vi "API Usage Examples.vi"() -> ()   [LabVIEW 2024, in "serenial.io-ase.example.lvlib"]
doc: "<B>A range of API usage examples for different scenarios.</B>"
uses:
  serenial.io-ase.example.lvlib
  serenial.io-ase/ase/ase.lvclass/ase.ctl
  Example Custom Regex/Example Custom Regex.lvclass
  serenial.io-ase/ase/Standard Output.ctl
  serenial.io-ase/ase/Did Exit.ctl
  serenial.io-ase/ase/Event References.ctl
  serenial.io-ase/ase/Standard Error.ctl
  serenial.io-ase/ase/Start Call (Command).vi
  serenial.io-ase/ase/Write Line to Std In .vi
  serenial.io-ase/ase/Start Call (Exe-Args).vi
  serenial.io-ase/ase/Start Call (Internal).vi
  serenial.io-ase/ase/Merge Call Library Errors.vi
  serenial.io-ase/ase/Write Data to Std In.vi
  serenial.io-ase/ase/Error Invalid ASE Handle.vi
  serenial.io-ase/ase/Error Empty Executable Name.vi
  serenial.io-ase/ase/Check Shared Library Version.vi
  serenial.io-ase/ase/Trim Whitespace.vi
  serenial.io-ase/ase/Error Internal Library Implementation Error.vi
  Example Custom ID/Example Custom ID.lvclass
  <vilib>/Utility/error.llb/Error Cluster From Error Code.vi
  serenial.io-ase/configuration/configuration.lvclass
  serenial.io-ase/ase/ase.lvclass
  C:/Users/marc/code/sift-streaming/labview/Sift/Dependencies/asynchronous-system-exec-v2.0.0/serenial.io-ase/configuration/configuration.lvclass
  C:/Users/marc/code/sift-streaming/labview/Sift/Dependencies/asynchronous-system-exec-v2.0.0/serenial.io-ase.example/Example Custom ID/Example Custom ID.lvclass
  C:/Users/marc/code/sift-streaming/labview/Sift/Dependencies/asynchronous-system-exec-v2.0.0/serenial.io-ase.example/Example Custom Regex/Example Custom Regex.lvclass
panel:
  out "Exit Code":i32
  out "error out":errorcluster
  out "Exit Code":i32
  out "error out":errorcluster
  out "Std Out":string caption="Std Out (regex split on numeric)"
  out "Exit Code":i32
  out "error out":errorcluster
  out "Std Out":string
  out "error out":errorcluster
  out "Std Out":string
  out "error out":errorcluster
  out "Std Out":string
  out "Exit Code":i32
  out "error out":errorcluster
  out "Std Out":string
  out "Exit Code":i32
  out "error out":errorcluster
  out "error out":errorcluster
  out "Exit Code":i32
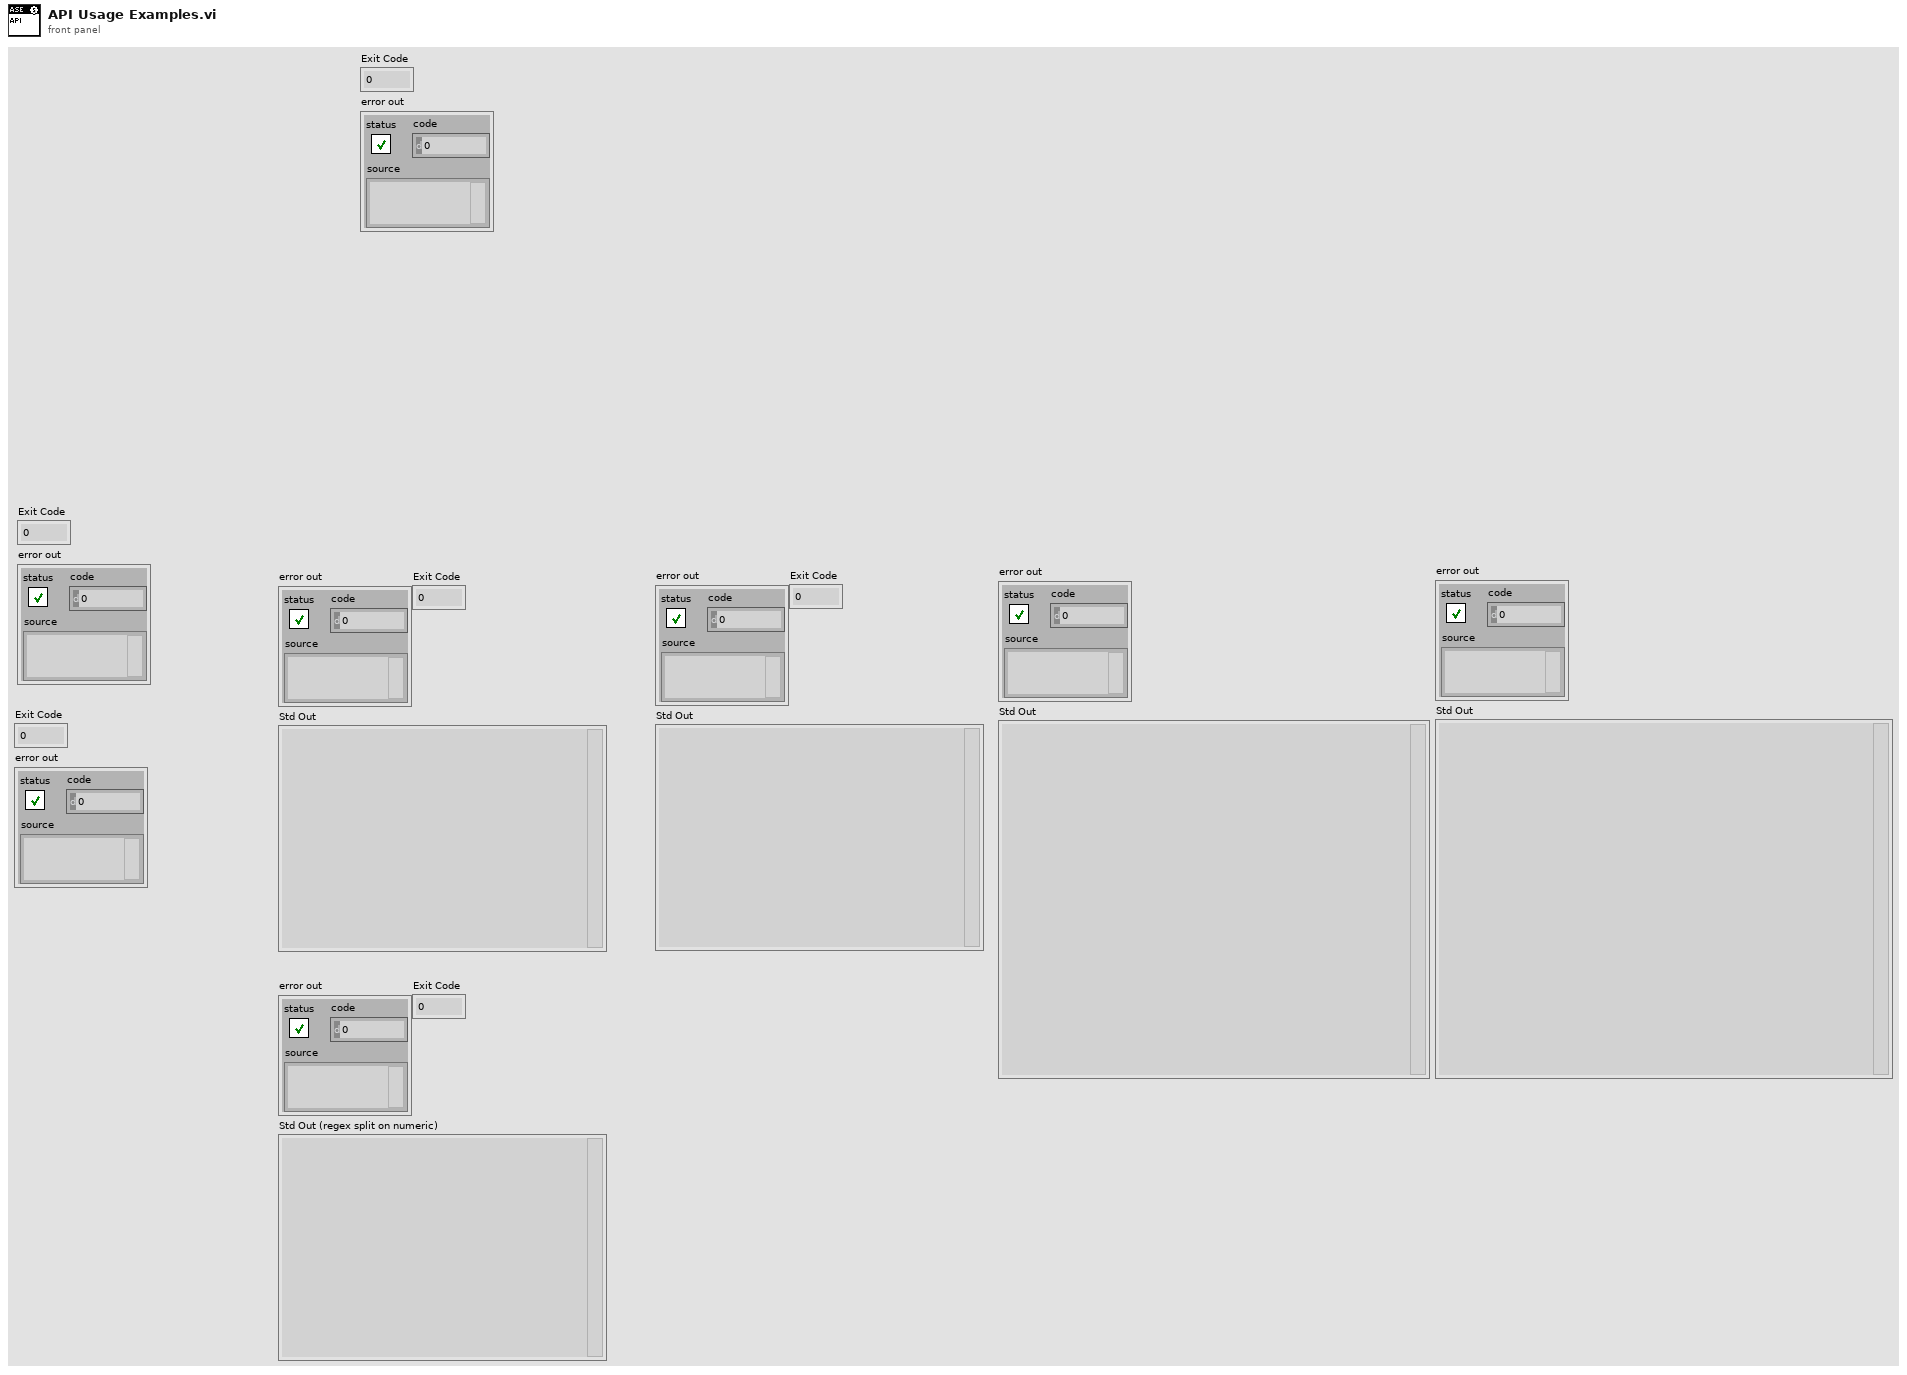
[diagram p1: front panel]
types:
  T1 = typedef "serenial.io-ase.lvlib/ase.lvclass/Event References.ctl" = cluster{"Standard Output":refnum<user-event>, "Standard Error":refnum<user-event>, "Did Exit":refnum<user-event>}
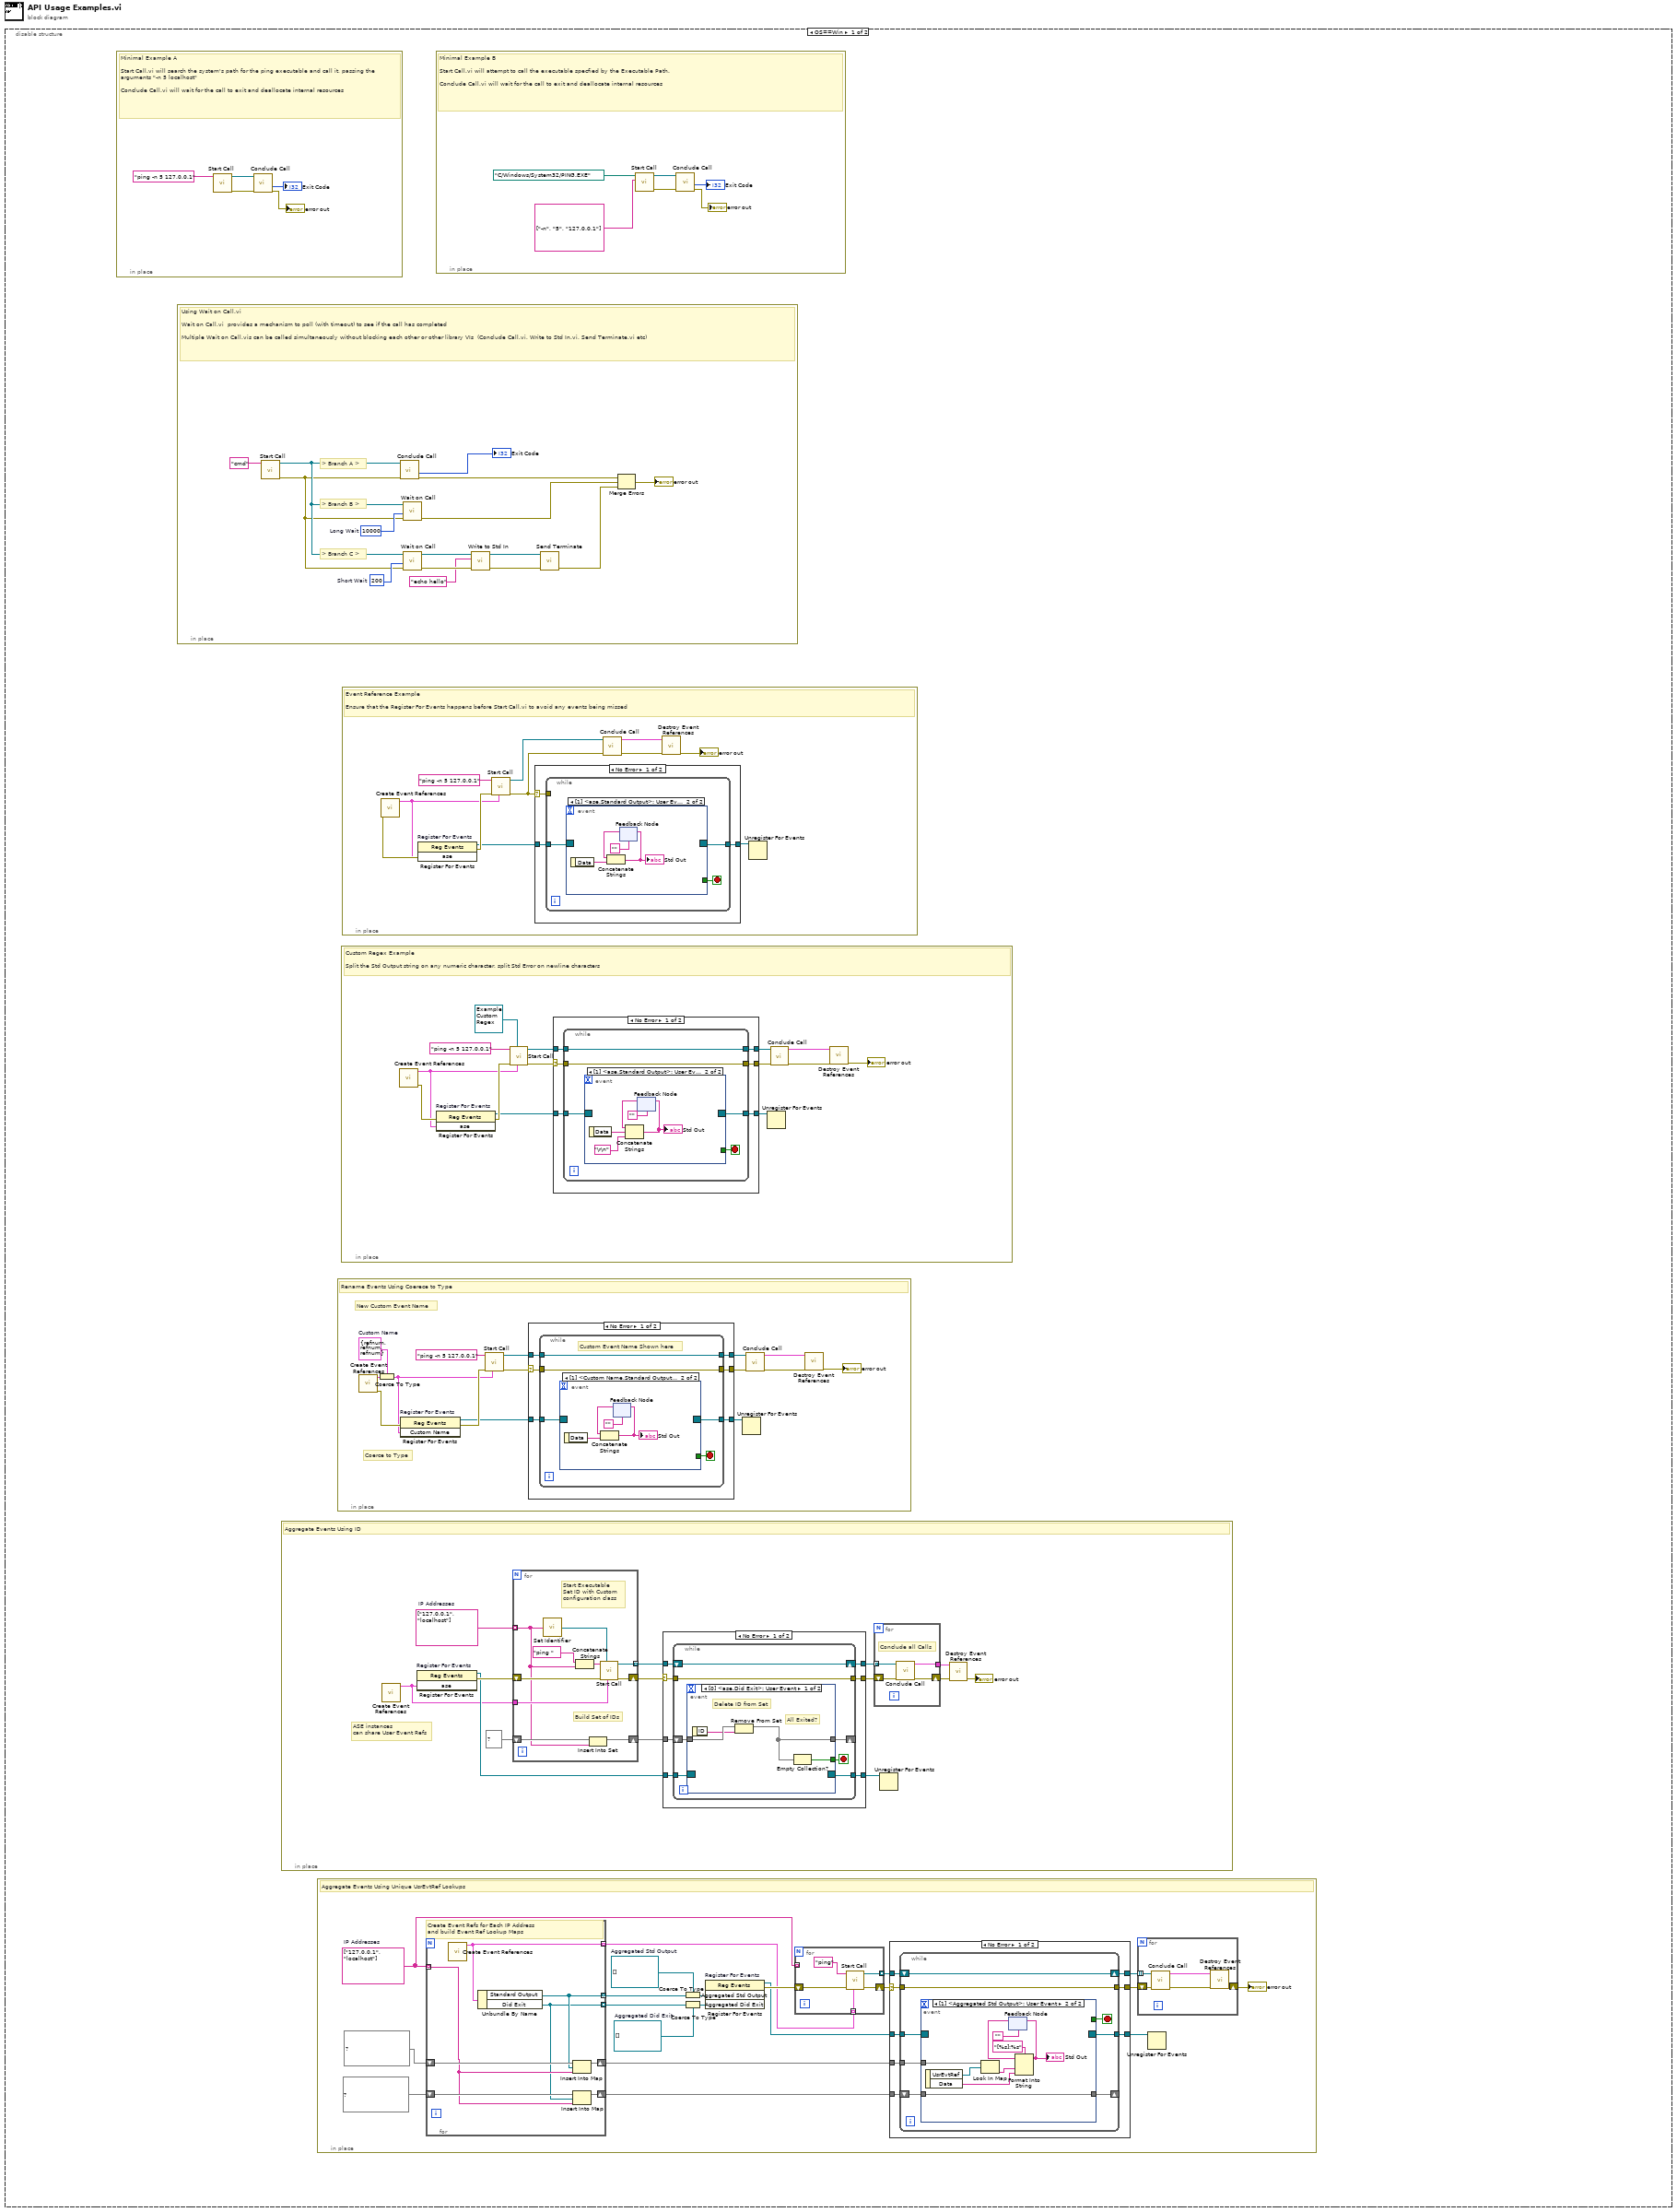
[diagram p0: block diagram]
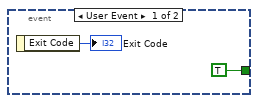
[diagram p2: hidden frame]
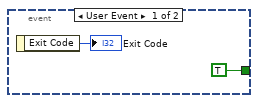
[diagram p4: hidden frame]
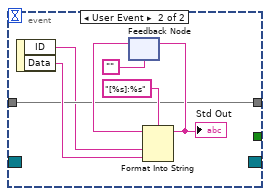
[diagram p6: hidden frame]
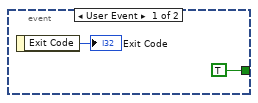
[diagram p8: hidden frame]
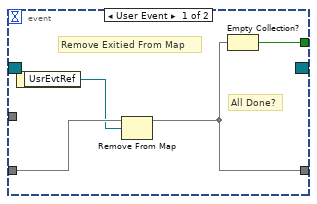
[diagram p10: hidden frame]
diagram:
  n1 = disable-structure shown="OS==Win" {
    frame condition #0 (active) {
      n2 = in-place {
        # "Minimal Example A\n\nStart Call.vi will search the system's path for the ping executable and call it, passing the arguments \"-n 5 localhost\"\n\nConclude Call.vi will wait for the call to exit and deallocate internal resources"
        n3 = call-poly "Start Call.vi"("Command"="ping -n 5 127.0.0.1" ("cmd")) -> ("error out"=w170:errorcluster, "New ASE Handle"=w169:refnum<class "ase.lvclass">)  [unwired: 9 in]
        n4 = call "Conclude Call.vi"("error in"=w170, "ASE Handle"=w169) -> ("error out"=→"error out":errorcluster, "Exit Code"=→"Exit Code":i32)  [unwired: 7 in, 1 out]
      }
      n5 = in-place {
        w162 = 200  # Short Wait
        w163 = 10000  # Long Wait
        # "> Branch C >"
        # "> Branch B >"
        # "> Branch A >"
        # "Using Wait on Call.vi\n\nWait on Call.vi  provides a mechanism to poll (with timeout) to see if the call has completed\n\nMultiple Wait on Call.vis can be called simultaneously without blocking each other or other library VIs  (Conclude Call.vi, Write to Std In.vi, Send Terminate.vi etc)"
        n6 = call-poly "Start Call.vi"("Command"="cmd" ("cmd")) -> ("error out"=w153:errorcluster, "New ASE Handle"=w156:refnum<class "ase.lvclass">)  [unwired: 9 in]
        n7 = call "Conclude Call.vi"("error in"=w153, "ASE Handle"=w156) -> ("error out"=w155:errorcluster, "Exit Code"=→"Exit Code":i32)  [unwired: 7 in, 1 out]
        n8 = call "Wait on Call.vi"("error in"=w153, "Timeout (ms)"=w163, "ASE Handle"=w156) -> ("error out"=w152:errorcluster)  [unwired: 6 in, 2 out]
        n9 = call "Wait on Call.vi"("error in"=w153, "Timeout (ms)"=w162, "ASE Handle"=w156) -> ("error out"=w160:errorcluster, "ASE Handle Duplicate"=w161:refnum<class "ase.lvclass">)  [unwired: 6 in, 1 out]
        n10 = call-poly "Write to Std In.vi"("error in"=w160, "Input"="echo hello", "ASE Handle"=w161) -> ("error out"=w157:errorcluster, "ASE Handle Duplicate"=w158:refnum<class "ase.lvclass">)  [unwired: 6 in, 1 out]
        n11 = call "Send Terminate.vi"("error in"=w157, "ASE Handle"=w158) -> ("error out"=w151:errorcluster)  [unwired: 7 in, 2 out]
        n12 = Merge Errors(w155, w152, w151) -> (→"error out":errorcluster)
      }
      n13 = in-place {
        w66 = string[] ["127.0.0.1", "localhost"]  # IP Addresses
        # "ASE instances\ncan share User Event Refs"
        # "Aggregate Events Using ID"
        n14 = call "Create Event References.vi"() -> ("ase"=w65:T1)  [unwired: 10 in, 1 out]
        n15 = register-events "Register For Events"(w65) -> (reference out=w70:refnum<event-registration>, error out=w73:errorcluster)  [unwired: 2 in]
        n16 = for {
          tunnel: [w82] -> w72 mode=indexing
          shift-right: [w81] -> w67
          shift-left: w73 -> [w83]
          tunnel: w65 -> [w80]
          tunnel: w66 -> [w74] mode=indexing
          shift-right: [w79] -> w63
          shift-left: set{string} {} ("Size: 0") -> [w78]
          # "Build Set of IDs"
          # "Start Executable\nSet ID with Custom \nconfiguration class"
          # "Use IP Address as ID"
          n17 = call "Set Identifier.vi"("Custom ID"=w74) -> ("Example Custom ID out"=w76:refnum<class "Example Custom ID.lvclass">)
          n18 = Concatenate Strings("ping ", w74) -> (w75:string)
          n19 = Insert Into Set(10:w74, 11:w78) -> (3:w79:set{string})  [unwired: 1 out]
          n20 = call-poly "Start Call.vi"("Event References"=w80, "Configuration"=w76, "error in"=w83, "Command"=w75) -> ("error out"=w81:errorcluster, "New ASE Handle"=w82:refnum<class "ase.lvclass">)  [unwired: 6 in]
        }
        n21 = case shown="No Error" w67 {
          selector: w67 -> [w88 w109]
          tunnel: w72 -> [w90 w110]
          tunnel: [w89 w110] -> w71
          tunnel: w70 -> [w87 w111]
          tunnel: [w86 w111] -> w69
          tunnel: [w85 w109] -> w68
          tunnel: w63 -> [w84 _]
          frame No Error {
            n22 = while {
              tunnel: w88 -> [w94]
              tunnel: w87 -> [w96]
              tunnel: [w95] -> w86
              tunnel: [w94] -> w85
              shift-right: [w91] -> _
              shift-left: w84 -> [w92]
              shift-right: [w97] -> w89
              shift-left: w90 -> [w97]
              stop <- w93 stop-if-true
              n23 = event shown="[0] <ase.Did Exit>: User Event" {
                selector: w96 -> [_ _]
                dyn-events: [_ _] -> w95
                timeout: _ -> [_ _]
                tunnel: [w100 _] -> w93
                tunnel: w92 -> [w101 w103]
                tunnel: [w99 w103] -> w91
                event User Event {
                  # "All Exited?"
                  # "Delete ID from Set"
                  n24 = event-data() -> ("ID"=w98:string)  [unwired: 1 in]
                  n25 = Remove From Set(10:w98, 11:w101) -> (3:w99:set{string})  [unwired: 1 out]
                  n26 = Empty Collection?(1:w99) -> (0:w100:bool)
                }
                event User Event {
                  n27 = event-data() -> ("ID"=w102:string, "Data"=w104:string)  [unwired: 1 in]
                  n28 = feedback #1("") -> (w107:string)
                  n29 = Format Into String(format string="[%s]:%s", initial string=w107, w102, w104) -> (resulting string=w106:string)  [unwired: 1 in, 1 out]
                  "Std Out" <- w106
                  n30 = feedback-in #1(w106) -> ()
                }
              }
            }
          }
          frame Error {
          }
        }
        n31 = for {
          tunnel: w71 -> [w115] mode=indexing
          shift-right: [w112] -> w60
          shift-left: w68 -> [w114]
          tunnel: [w113] -> w62
          # "Conclude all Calls"
          n32 = call "Conclude Call.vi"("error in"=w114, "ASE Handle"=w115) -> ("error out"=w112:errorcluster, "Event References"=w113:T1)  [unwired: 7 in, 1 out]
        }
        n33 = Unregister For Events(event registration refnum=w69) -> ()  [unwired: 1 in, 1 out]
        n34 = call "Destroy Event References.vi"("error in"=w60, "Event References"=w62) -> ("error out"=→"error out":errorcluster)  [unwired: 9 in]
      }
      n35 = in-place {
        w171 = string[] ["127.0.0.1", "localhost"]  # IP Addresses
        w173 = refnum<user-event>[] []  # Aggregated Did Exit
        w172 = refnum<user-event>[] []  # Aggregated Std Output
        # "Aggregate Events Using Unique UsrEvtRef Lookups"
        n36 = for {
          tunnel: w171 -> [w202] mode=indexing
          shift-right: [w206] -> w178
          shift-left: map{refnum<user-event>, string} {} ("map out") -> [w207]
          shift-right: [w204] -> w177
          shift-left: map{refnum<user-event>, string} {} ("set out") -> [w203]
          tunnel: [w208] -> w179 mode=indexing
          tunnel: [w205] -> w181 mode=indexing
          tunnel: [w201] -> w180 mode=indexing
          # "Create Event Refs for Each IP Address\nand build Event Ref Lookup Maps"
          n37 = call "Create Event References.vi"() -> ("ase"=w208:T1)  [unwired: 10 in, 1 out]
          n38 = Unbundle By Name(w208) -> ("Standard Output"=w205:refnum<user-event>, "Did Exit"=w201:refnum<user-event>)
          n39 = Insert Into Map(map in=w207, key=w205, value=w202) -> (map out=w206:map{refnum<user-event>, string})  [unwired: 2 out]
          n40 = Insert Into Map(map in=w203, key=w201, value=w202) -> (map out=w204:map{refnum<user-event>, string})  [unwired: 2 out]
        }
        n41 = Coerce To Type(0:w181, 1:w172) -> (2:w175:refnum<user-event>[])
        n42 = Coerce To Type(0:w180, 1:w173) -> (2:w174:refnum<user-event>[])
        n43 = register-events "Register For Events"(w175, w174) -> (reference out=w187:refnum<event-registration>, error out=w190:errorcluster)  [unwired: 2 in]
        n44 = for {
          tunnel: [w199] -> w189 mode=indexing
          shift-right: [w198] -> w184
          shift-left: w190 -> [w200]
          tunnel: w179 -> [w197] mode=indexing
          tunnel: w171 -> [_] mode=indexing
          n45 = call-poly "Start Call.vi"("Event References"=w197, "error in"=w200, "Command"="ping") -> ("error out"=w198:errorcluster, "New ASE Handle"=w199:refnum<class "ase.lvclass">)  [unwired: 7 in]
        }
        n46 = case shown="No Error" w184 {
          selector: w184 -> [w214 w238]
          tunnel: w189 -> [w216 w239]
          tunnel: [w215 w239] -> w188
          tunnel: w187 -> [w213 w240]
          tunnel: [w212 w240] -> w186
          tunnel: [w211 w238] -> w185
          tunnel: w178 -> [w210 _]
          tunnel: w177 -> [w209 _]
          frame No Error {
            n47 = while {
              tunnel: w214 -> [w221]
              tunnel: w213 -> [w223]
              tunnel: [w222] -> w212
              tunnel: [w221] -> w211
              tunnel: w210 -> [w219]
              shift-right: [w217] -> _
              shift-left: w209 -> [w218]
              shift-right: [w224] -> w215
              shift-left: w216 -> [w224]
              stop <- w220 stop-if-true
              n48 = event shown="[1] <Aggregated Std Output>: User Event" {
                selector: w223 -> [_ _]
                dyn-events: [_ _] -> w222
                timeout: _ -> [_ _]
                tunnel: [w226 _] -> w220
                tunnel: w219 -> [_ w236]
                tunnel: w218 -> [w228 w230]
                tunnel: [w225 w230] -> w217
                event User Event {
                  # "All Done?"
                  # "Remove Exitied From Map"
                  n49 = event-data() -> ("UsrEvtRef"=w227:refnum<user-event>)  [unwired: 1 in]
                  n50 = Remove From Map(10:w227, 11:w228) -> (3:w225:map{refnum<user-event>, string})  [unwired: 2 out]
                  n51 = Empty Collection?(1:w225) -> (0:w226:bool)
                }
                event User Event {
                  n52 = event-data() -> ("UsrEvtRef"=w235:refnum<user-event>, "Data"=w229:string)  [unwired: 1 in]
                  n53 = Look In Map(map=w236, key=w235) -> (value=w234:string)  [unwired: 1 in, 1 out]
                  n54 = feedback #2("") -> (w233:string)
                  n55 = Format Into String(format string="[%s]:%s", initial string=w233, w234, w229) -> (resulting string=w232:string)  [unwired: 1 in, 1 out]
                  "Std Out" <- w232
                  n56 = feedback-in #2(w232) -> ()
                }
              }
            }
          }
          frame Error {
          }
        }
        n57 = for {
          tunnel: w188 -> [w195] mode=indexing
          shift-right: [w191] -> w183
          shift-left: w185 -> [w194]
          n58 = call "Conclude Call.vi"("error in"=w194, "ASE Handle"=w195) -> ("error out"=w193:errorcluster, "Event References"=w192:T1)  [unwired: 7 in, 1 out]
          n59 = call "Destroy Event References.vi"("error in"=w193, "Event References"=w192) -> ("error out"=w191:errorcluster)  [unwired: 9 in]
        }
        "error out" <- w183
        n60 = Unregister For Events(event registration refnum=w186) -> ()  [unwired: 1 in, 1 out]
      }
      n61 = in-place {
        w117 = T1 {"Standard Output"=refnum, "Standard Error"=refnum, "Did Exit"=refnum}  # Custom Name
        # "New Custom Event Name"
        # "Coerce to Type"
        # "Rename Events Using Coerece to Type"
        n62 = call "Create Event References.vi"() -> ("error out"=w128:errorcluster, "ase"=w127:T1)  [unwired: 10 in]
        n63 = Coerce To Type(0:w127, 1:w117) -> (2:w116:T1)
        n64 = register-events "Register For Events"(error in=w128, w116) -> (reference out=w124:refnum<event-registration>, error out=w130:errorcluster)  [unwired: 1 in]
        n65 = call-poly "Start Call.vi"("Event References"=w116, "error in"=w130, "Command"="ping -n 5 127.0.0.1" ("cmd")) -> ("error out"=w121:errorcluster, "New ASE Handle"=w126:refnum<class "ase.lvclass">)  [unwired: 7 in]
        n66 = case shown="No Error" w121 {
          selector: w121 -> [w134 w148]
          tunnel: w126 -> [w136 w149]
          tunnel: [w135 w149] -> w125
          tunnel: w124 -> [w133 w150]
          tunnel: [w132 w150] -> w123
          tunnel: [w131 w148] -> w122
          frame No Error {
            n67 = while {
              tunnel: w136 -> [w141]
              tunnel: [w141] -> w135
              tunnel: w134 -> [w138]
              tunnel: w133 -> [w140]
              tunnel: [w139] -> w132
              tunnel: [w138] -> w131
              stop <- w137 stop-if-true
              # "Custom Event Name Shown here"
              n68 = event shown="[1] <Custom Name.Standard Output>: User Event" {
                selector: w140 -> [_ _]
                dyn-events: [_ _] -> w139
                timeout: _ -> [_ _]
                tunnel: [TRUE _] -> w137
                event User Event {
                  n69 = event-data() -> ("Exit Code"=→"Exit Code":i32)  [unwired: 1 in]
                }
                event User Event {
                  n70 = event-data() -> ("Data"=w147:string)  [unwired: 1 in]
                  n71 = feedback #3("") -> (w145:string)
                  n72 = Concatenate Strings(w145, w147) -> (w146:string)
                  "Std Out" <- w146
                  n73 = feedback-in #3(w146) -> ()
                }
              }
            }
          }
          frame Error {
          }
        }
        n74 = Unregister For Events(event registration refnum=w123) -> ()  [unwired: 1 in, 1 out]
        n75 = call "Conclude Call.vi"("error in"=w122, "ASE Handle"=w125) -> ("error out"=w120:errorcluster, "Event References"=w119:T1)  [unwired: 7 in, 1 out]
        n76 = call "Destroy Event References.vi"("error in"=w120, "Event References"=w119) -> ("error out"=→"error out":errorcluster)  [unwired: 9 in]
      }
      n77 = in-place {
        # "Custom Regex Example\n\nSplit the Std Output string on any numeric character, split Std Error on newline characters"
        n78 = call "Create Event References.vi"() -> ("error out"=w12:errorcluster, "ase"=w11:T1)  [unwired: 10 in]
        n79 = register-events "Register For Events"(error in=w12, w11) -> (reference out=w8:refnum<event-registration>, error out=w14:errorcluster)  [unwired: 1 in]
        n80 = call-poly "Start Call.vi"("Event References"=w11, "Configuration"=refnum<class "Example Custom Regex.lvclass"> refnum ("serenial.io-ase.example.lvlib:Example Configuration.lvclass"), "error in"=w14, "Command"="ping -n 5 127.0.0.1" ("cmd")) -> ("error out"=w5:errorcluster, "New ASE Handle"=w10:refnum<class "ase.lvclass">)  [unwired: 6 in]
        n81 = case shown="No Error" w5 {
          selector: w5 -> [w18 w33]
          tunnel: w10 -> [w20 w34]
          tunnel: [w19 w34] -> w9
          tunnel: w8 -> [w17 w35]
          tunnel: [w16 w35] -> w7
          tunnel: [w15 w33] -> w6
          frame No Error {
            n82 = while {
              tunnel: w20 -> [w25]
              tunnel: [w25] -> w19
              tunnel: w18 -> [w22]
              tunnel: w17 -> [w24]
              tunnel: [w23] -> w16
              tunnel: [w22] -> w15
              stop <- w21 stop-if-true
              n83 = event shown="[1] <ase.Standard Output>: User Event" {
                selector: w24 -> [_ _]
                dyn-events: [_ _] -> w23
                timeout: _ -> [_ _]
                tunnel: [TRUE _] -> w21
                event User Event {
                  n84 = event-data() -> ("Exit Code"=→"Exit Code":i32)  [unwired: 1 in]
                }
                event User Event {
                  n85 = event-data() -> ("Data"=w29:string)  [unwired: 1 in]
                  n86 = feedback #4("") -> (w31:string)
                  n87 = Concatenate Strings(w31, w29, "\r\n" ("string")) -> (w32:string)
                  "Std Out" <- w32
                  n88 = feedback-in #4(w32) -> ()
                }
              }
            }
          }
          frame Error {
          }
        }
        n89 = Unregister For Events(event registration refnum=w7) -> ()  [unwired: 1 in, 1 out]
        n90 = call "Conclude Call.vi"("error in"=w6, "ASE Handle"=w9) -> ("error out"=w4:errorcluster, "Event References"=w3:T1)  [unwired: 7 in, 1 out]
        n91 = call "Destroy Event References.vi"("error in"=w4, "Event References"=w3) -> ("error out"=→"error out":errorcluster)  [unwired: 9 in]
      }
      n92 = in-place {
        # "Event Reference Example\n\nEnsure that the Register For Events happens before Start Call.vi to avoid any events being missed"
        n93 = call "Create Event References.vi"() -> ("error out"=w44:errorcluster, "ase"=w43:T1)  [unwired: 10 in]
        n94 = register-events "Register For Events"(error in=w44, w43) -> (reference out=w42:refnum<event-registration>, error out=w46:errorcluster)  [unwired: 1 in]
        n95 = call-poly "Start Call.vi"("Event References"=w43, "error in"=w46, "Command"="ping -n 5 127.0.0.1" ("cmd")) -> ("error out"=w36:errorcluster, "New ASE Handle"=w37:refnum<class "ase.lvclass">)  [unwired: 7 in]
        n96 = case shown="No Error" w36 {
          selector: w36 -> [w49 _]
          tunnel: w42 -> [w48 w59]
          tunnel: [w47 w59] -> w41
          frame No Error {
            n97 = while {
              tunnel: w49 -> [_]
              tunnel: w48 -> [w52]
              tunnel: [w51] -> w47
              stop <- w50 stop-if-true
              n98 = event shown="[1] <ase.Standard Output>: User Event" {
                selector: w52 -> [_ _]
                dyn-events: [_ _] -> w51
                timeout: _ -> [_ _]
                tunnel: [TRUE _] -> w50
                event User Event {
                  n99 = event-data() -> ("Exit Code"=→"Exit Code":i32)  [unwired: 1 in]
                }
                event User Event {
                  n100 = event-data() -> ("Data"=w58:string)  [unwired: 1 in]
                  n101 = feedback #5("") -> (w56:string)
                  n102 = Concatenate Strings(w56, w58) -> (w57:string)
                  "Std Out" <- w57
                  n103 = feedback-in #5(w57) -> ()
                }
              }
            }
          }
          frame Error {
          }
        }
        n104 = call "Conclude Call.vi"("error in"=w36, "ASE Handle"=w37) -> ("error out"=w40:errorcluster, "Event References"=w39:T1)  [unwired: 7 in, 1 out]
        n105 = call "Destroy Event References.vi"("error in"=w40, "Event References"=w39) -> ("error out"=→"error out":errorcluster)  [unwired: 9 in]
        n106 = Unregister For Events(event registration refnum=w41) -> ()  [unwired: 1 in, 1 out]
      }
      n107 = in-place {
        # "Minimal Example B\n\nStart Call.vi will attempt to call the executable specfied by the Executable Path.\n\nConclude Call.vi will wait for the call to exit and deallocate internal resources"
        n108 = call-poly "Start Call.vi"("Arguments (Default: Empty)"=string[] ["-n", "5", "127.0.0.1"], "Executable Path"=path "C:/Windows/System32/PING.EXE") -> ("error out"=w246:errorcluster, "New ASE Handle"=w245:refnum<class "ase.lvclass">)  [unwired: 8 in]
        n109 = call "Conclude Call.vi"("error in"=w246, "ASE Handle"=w245) -> ("error out"=→"error out":errorcluster, "Exit Code"=→"Exit Code":i32)  [unwired: 7 in, 1 out]
      }
    }
    frame condition #1 {
      # "These examples will work on other platforms but the ping executable needs to be supplied a \"ping count\"  with option -\"c\"  instead of option \"-n\""
    }
  }
